vi "Step_Sequence_byteread.vi"(6 "Polarity":bool, 7 "Direction in":bool, 8 "error in":errorcluster, 9 "Steps in":i32(slide)=1 min=1 max=10000 step=1 scale=1.0..10000.0, 10 "Step Time (us) in":i32(slide)=100 min=100 max=10000 step=10 scale=100.0..10000.0, 11 "VISA resource name":refnum<visa-resource-name>) -> (0 "error out":errorcluster, 3 "VISA out":refnum<visa-resource-name>)   [LabVIEW 2023]
uses:
  <vilib>/Instr/_visa.llb/Select Event Type.ctl
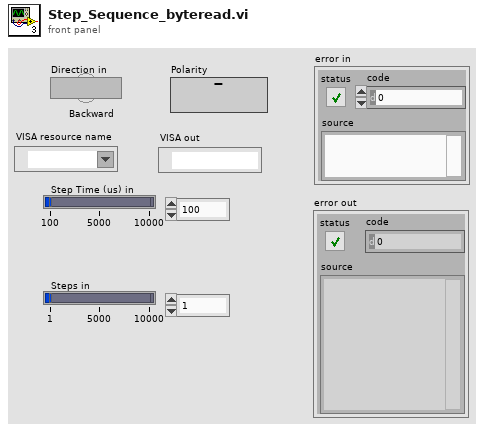
[diagram p1: front panel]
types:
  T1 = typedef "Select Event Type.ctl" = u32
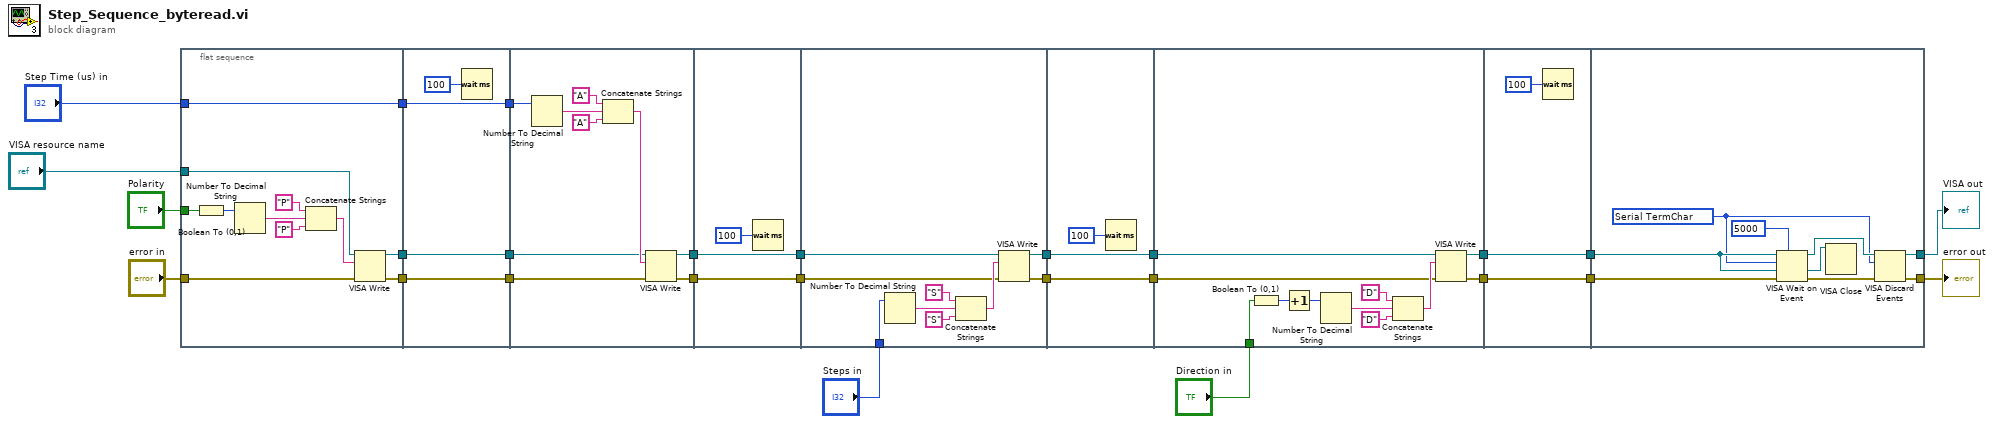
[diagram p0: block diagram]
diagram:
  n1 = flat-sequence {
    tunnel: "VISA resource name" -> [w29]
    tunnel: "Step Time (us) in" -> [w37]
    tunnel: "error in" -> [w33]
    tunnel: [w32] -> w6
    tunnel: [w37] -> w5
    tunnel: [w30] -> w4
    tunnel: "Polarity" -> [w28]
    tunnel: [w41] -> w9
    tunnel: [w40] -> w8
    tunnel: [w39] -> w7
    tunnel: w6 -> [w41]
    tunnel: w5 -> [w40]
    tunnel: w4 -> [w39]
    tunnel: [w46] -> w26
    tunnel: [w42] -> w10
    tunnel: w9 -> [w48]
    tunnel: w8 -> [w44]
    tunnel: w7 -> [w43]
    tunnel: [w52] -> w25
    tunnel: w26 -> [w52]
    tunnel: [w51] -> w11
    tunnel: w10 -> [w51]
    tunnel: w25 -> [w59]
    tunnel: [w58] -> w23
    tunnel: [w56] -> w24
    tunnel: "Steps in" -> [w55]
    tunnel: w11 -> [w54]
    tunnel: [w65] -> w22
    tunnel: [w64] -> w21
    tunnel: w24 -> [w64]
    tunnel: w23 -> [w65]
    tunnel: [w76] -> w20
    tunnel: [w75] -> w19
    tunnel: "Direction in" -> [w68]
    tunnel: w22 -> [w66]
    tunnel: w21 -> [w67]
    tunnel: w20 -> [w79]
    tunnel: w19 -> [w78]
    tunnel: [w79] -> w18
    tunnel: [w78] -> w17
    tunnel: w17 -> [w85]
    tunnel: w18 -> [w88]
    tunnel: [w81] -> w2
    tunnel: [w80] -> w1
    frame #0 {
      n2 = Boolean To (0,1)(Boolean=w28) -> (0, 1=w27:i16)
      n3 = Number To Decimal String(number=w27) -> (decimal integer string=w34:string)  [unwired: 1 in]
      n4 = Concatenate Strings("P" ("write buffer"), w34, "P" ("string")) -> (w35:string)
      n5 = VISA Write(VISA resource name=w29, write buffer=w35, error in (no error)=w33) -> (VISA resource name out=w30:refnum<visa-resource-name>, error out=w32:errorcluster)  [unwired: 1 out]
    }
    frame #1 {
      n6 = Wait (ms)(milliseconds to wait=u32 100) -> ()  [unwired: 1 out]
    }
    frame #2 {
      n7 = Number To Decimal String(number=w44) -> (decimal integer string=w45:string)  [unwired: 1 in]
      n8 = Concatenate Strings("A" ("write buffer"), w45, "A" ("string")) -> (w47:string)
      n9 = VISA Write(VISA resource name=w43, write buffer=w47, error in (no error)=w48) -> (VISA resource name out=w42:refnum<visa-resource-name>, error out=w46:errorcluster)  [unwired: 1 out]
    }
    frame #3 {
      n10 = Wait (ms)(milliseconds to wait=u32 100) -> ()  [unwired: 1 out]
    }
    frame #4 {
      n11 = Number To Decimal String(number=w55) -> (decimal integer string=w57:string)  [unwired: 1 in]
      n12 = Concatenate Strings("S" ("write buffer"), w57, "S" ("string")) -> (w60:string)
      n13 = VISA Write(VISA resource name=w54, write buffer=w60, error in (no error)=w59) -> (VISA resource name out=w56:refnum<visa-resource-name>, error out=w58:errorcluster)  [unwired: 1 out]
    }
    frame #5 {
      n14 = Wait (ms)(milliseconds to wait=u32 100) -> ()  [unwired: 1 out]
    }
    frame #6 {
      n15 = Boolean To (0,1)(Boolean=w68) -> (0, 1=w71:i16)
      n16 = Increment(x=w71) -> (x+1=w70:i16)
      n17 = Number To Decimal String(number=w70) -> (decimal integer string=w69:string)  [unwired: 1 in]
      n18 = Concatenate Strings("D" ("write buffer"), w69, "D" ("string")) -> (w73:string)
      n19 = VISA Write(VISA resource name=w67, write buffer=w73, error in (no error)=w66) -> (VISA resource name out=w75:refnum<visa-resource-name>, error out=w76:errorcluster)  [unwired: 1 out]
    }
    frame #7 {
      n20 = Wait (ms)(milliseconds to wait=u32 100) -> ()  [unwired: 1 out]
    }
    frame #8 {
      w82 = T1 1073684516 items=["Service Request"=1073684491, "Trigger"=3221168138, "Clear"=1073684493, "VXI Signal"=1073684512, "VXI/VME Interrupt"=3221168161, "VXI/VME Sysfail"=1073684509, "VXI/VME Sysreset"=1073684510, "GPIB CIC"=1073684498, "GPIB Talk"=1073684499, "GPIB Listen"=1073684500, "PXI Interrupt"=1073684514, "Serial Break"=1073684515, "Serial TermChar"=1073684516, "Serial CTS"=1073684521, "Serial DSR"=1073684522, "Serial DCD"=1073684524, "Serial RI"=1073684526, "Serial Character"=1073684533, "USB Interrupt"=1073684535, "All Enabled"=1073709055] ("Event Type")
      n21 = VISA Wait on Event(7:u32 5000 ("timeout (0)"), 8:w88, 9:w85, 10:w82, 11:w85) -> (0:w83:errorcluster, 1:w86:refnum<visa-resource-name>, 3:w84:refnum<visa-resource-name>)  [unwired: 1 out]
      n22 = VISA Close(VISA resource name=w86) -> ()  [unwired: 1 in, 1 out]
      n23 = VISA Discard Events(8:w83, 10:w82, 11:w84) -> (0:w80:errorcluster, 3:w81:refnum<visa-resource-name>)  [unwired: 1 in]
    }
  }
  "VISA out" <- w2
  "error out" <- w1
